vi "Read H2O Concentration DBL.vi"(8 "error in":errorcluster, 10 "Source":string, 11 "IRead Water Concentration in":refnum<class "IRead H2O Concentration.lvclass">) -> (0 "error out":errorcluster, 1 "Time Stamp":timestamp format="%<%x %.3X>T", 2 "H2O Concentration":dbl, 3 "IRead Water Concentration out":refnum<class "IRead H2O Concentration.lvclass">)   [LabVIEW 2024, in "IRead H2O Concentration.lvclass"]
uses:
  IRead H2O Concentration.lvclass
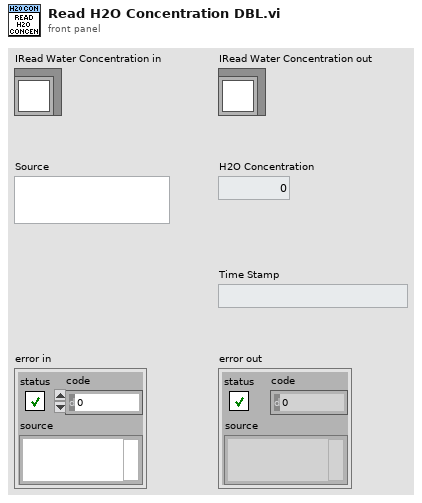
[diagram p1: front panel]
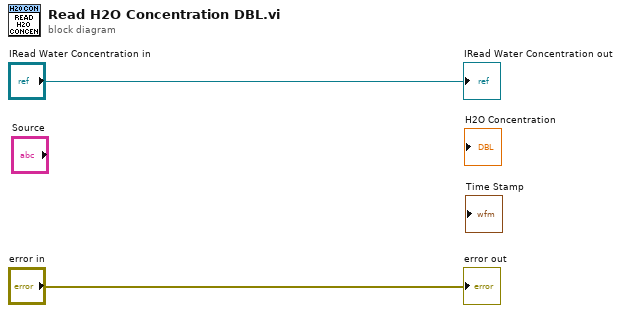
[diagram p0: block diagram]
diagram:
  "error out" <- "error in"
  "IRead Water Concentration out" <- "IRead Water Concentration in"
